vi "Synthesizer.vi"(7 "Status (F) (F: Off, T: On)":bool, 8 "error in (no error)":errorcluster) -> (0 "error out":errorcluster, 2 "Power":dbl, 3 "Frequency (GHz)":dbl)   [LabVIEW 2019, in "ACSVcontrol-driver.lvlib"]
doc: "Set synthesizer (micorwaves) on or off. This VI is not yet finished and is missing some possibilities."
uses:
  ACSVcontrol-driver.lvlib
  Private/Type definitions/Status.ctl
  Private/Type definitions/Command.ctl
  Private/Type definitions/Instruction.ctl
  Private/Globals.vi
  <vilib>/Utility/error.llb/Error Cluster From Error Code.vi
  <vilib>/ErrorRing/Error Ring.xnode
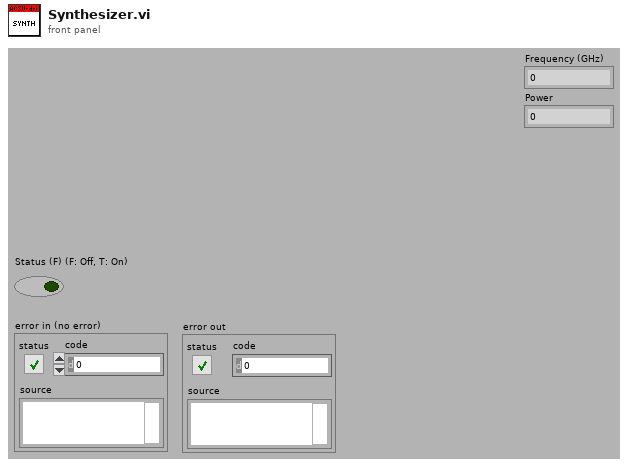
[diagram p1: front panel]
types:
  T1 = typedef "ACSVcontrol-driver.lvlib/Status.ctl" = enum16{"waiting", "processing", "error command", "Set_PJVS-Done", "Set_Mux-Done", "Set_Mux-Error", "Set_57XX-Done", "Set_57XX-Error", "Set_Gen-Done", "Set_Gen-Error", "Set_Synthesizer-Done", "Set_Synthesizer-Error", "Read_Nano-Done", "Read_Sampler-Done", "Read_Sampler-Error", "Read_Sensors-Done"}
  T2 = typedef "ACSVcontrol-driver.lvlib/Command.ctl" = enum16{"Set_PJVS", "Set_Mux", "Set_57XX", "Set_Gen", "Set_Synthesizer", "Read_Nulldetector", "Read_Sampler", "Read_Sensors"}
  T3 = typedef "ACSVcontrol-driver.lvlib/Instruction.ctl" = enum16{"dummy - do not use", "Send Command", "Read Result", "Ask Status"}
  T4 = typedef "ACSVcontrol-driver.lvlib/Timeouts.ctl" = cluster{"TCP Read & Write (ms)":i32, "Sensors readout":i32, "PJVS setup":i32, "Nullmeter readout":i32, "Multiplexer setup":i32, "57XX setup":i32, "Generator setup":i32, "Synthesizer setup":i32, "Sampler readout":i32}
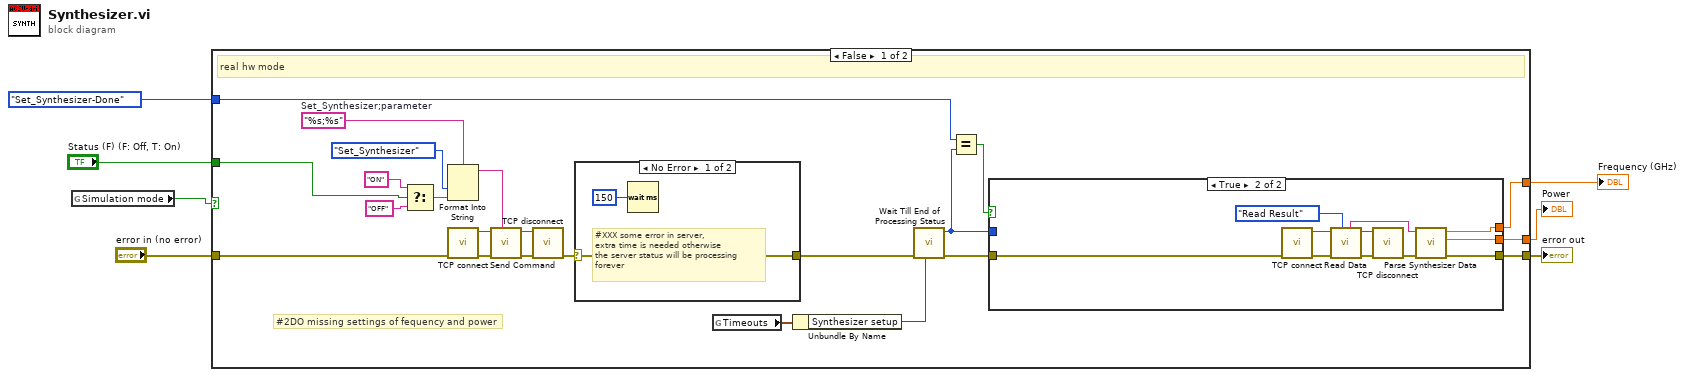
[diagram p0: block diagram]
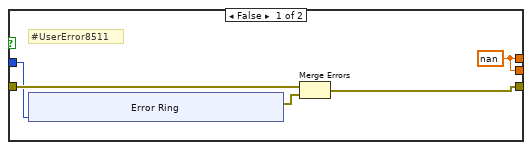
[diagram p3: hidden frame]
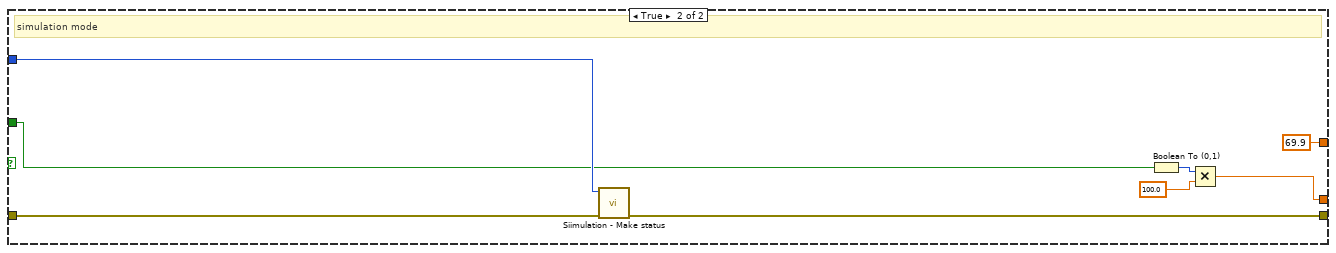
[diagram p4: hidden frame]
diagram:
  n1 = global read "Globals.vi" "Simulation mode"() -> (w2:bool)
  n2 = case shown="False" w2 {
    tunnel: "error in (no error)" -> [w27 w62]
    tunnel: [w19 69.9 ("Frequency (GHz)")] -> w6
    tunnel: [w18 w57] -> w5
    tunnel: [w17 w64] -> w4
    tunnel: Status."Set_Synthesizer-Done" ("x") -> [w9 w63]
    tunnel: "Status (F) (F: Off, T: On)" -> [w8 w60]
    frame False {
      w30 = "%s;%s"  # Set_Synthesizer;parameter
      # "#2DO missing settings of fequency and power"
      # "real hw mode"
      n3 = Select(t="ON" ("format string"), s=w8, f="OFF" ("format string")) -> (s? t:f=w28:string)
      n4 = Format Into String(format string=w30, Command."Set_Synthesizer" ("Command"), w28) -> (resulting string=w14:string)  [unwired: 2 in, 1 out]
      n5 = call "TCP connect.vi"("error in (no error)"=w27) -> ("error out"=w24:errorcluster, "connection ID"=w23:refnum<k5>)  [unwired: 9 in]
      n6 = call "Send Command.vi"("Command"=w14, "error in (no error)"=w24, "connection ID"=w23) -> ("error out"=w25:errorcluster, "connection ID out"=w26:refnum<k5>)  [unwired: 7 in]
      n7 = call "TCP disconnect.vi"("error in (no error)"=w25, "connection ID"=w26) -> ("error out"=w12:errorcluster)  [unwired: 9 in]
      n8 = case shown="No Error" w12 {
        selector: w12 -> [w31 w33]
        tunnel: [w31 w33] -> w11
        frame No Error {
          # "#XXX some error in server,\nextra time is needed otherwise\nthe server status will be processing\nforever"
          n9 = Wait (ms)(milliseconds to wait=u32 150) -> ()  [unwired: 1 out]
        }
        frame Error {
        }
      }
      n10 = global read "Globals.vi" "Timeouts"() -> (w15:T4)
      n11 = Unbundle By Name(w15) -> ("Synthesizer setup"=w16:i32)
      n12 = call "Wait Till End of Processing Status.vi"("Loop Timeout (ms) (5000)"=w16, "error in (no error)"=w11) -> ("error out"=w22:errorcluster, "Last Status"=w20:T1)  [unwired: 8 in]
      n13 = Equal?(x=w9, y=w20) -> (x = y?=w21:bool)
      n14 = case shown="True" w21 {
        tunnel: w22 -> [w38 w54]
        tunnel: w20 -> [w37 _]
        tunnel: [w35 w50] -> w19
        tunnel: [w35 w49] -> w18
        tunnel: [w34 w48] -> w17
        frame False {
          w35 = nan ("Frequency (GHz)")
          # "#UserError8511"
          n15 = xnode "Error Ring"("parameter 0"=w37) -> ("error out"=w36:errorcluster)
          n16 = Merge Errors(w38, w36) -> (w34:errorcluster)
        }
        frame True {
          n17 = call "TCP connect.vi"("error in (no error)"=w54) -> ("error out"=w53:errorcluster, "connection ID"=w52:refnum<k5>)  [unwired: 9 in]
          n18 = call "Read Data.vi"("Instruction"=Instruction."Read Result", "error in (no error)"=w53, "connection ID"=w52) -> ("error out"=w56:errorcluster, "connection ID out"=w55:refnum<k5>, "Data"=w46:string)  [unwired: 6 in]
          n19 = call "TCP disconnect.vi"("error in (no error)"=w56, "connection ID"=w55) -> ("error out"=w51:errorcluster)  [unwired: 9 in]
          n20 = call "Parse Synthesizer Data.vi"("error in"=w51, "Data"=w46) -> ("error out"=w48:errorcluster, "Power"=w49:dbl, "Frequency (GHz)"=w50:dbl)  [unwired: 7 in]
        }
      }
    }
    frame True {
      # "simulation mode"
      n21 = call "Siimulation - Make status.vi"("error in (no error)"=w62, "Status"=w63) -> ("error out"=w64:errorcluster)  [unwired: 8 in, 1 out]
      n22 = Boolean To (0,1)(Boolean=w60) -> (0, 1=w59:i16)
      n23 = Multiply(x=w59, y=100.0 ("Power")) -> (x*y=w57:dbl)
    }
  }
  "error out" <- w4
  "Frequency (GHz)" <- w6
  "Power" <- w5
